vi "Oscilloscope.vi"() -> ()   [LabVIEW 2011]
uses:
  <vilib>/Analysis/5stat.llb/RMS (DBL).vi
  <vilib>/express/express analysis/Spectral/Block/exnSpectralBlock spectral measurements peak poly.vi
  <vilib>/express/express analysis/Spectral/Block/exnSpectralBlock spectral measurements peak DDT.vi
  <vilib>/express/express analysis/Spectral/XNode/ExpressSpectralMeasurementsBlockNode.xnode
  <vilib>/Analysis/NI_AALPro.lvlib
panel:
  in  "OK Button 3":bool
  out "Peak":dbl format="%#_3gV"
  in  "Duty Cycle (%)":dbl(knob)=50.0 scale=0.0..100.0
  out "Recorded Time":dbl format="%#.3f"
  in  "Save File":bool
  in  "Tab Control":enum32{"Waveform", "FFT"}(tab)
  out "Waveform":waveform(dbl)(graph) caption="Sine"
  in  "Position":ext(knob) scale=-5.0..5.0
  in  "OK Button":bool
  in  "Trigger":bool
  in  "Save Waveform":bool
  out "FFT":dynamicdata(graph) caption="FFT - (Peak)"
  in  "Scale":bool caption="Linear/Log"
  in  "FFT X reset":bool
  in  "Save FFT":bool
  in  "Offset RST":bool
  in  "Offset":dbl(knob) scale=-5.0..5.0
  out "Frequency":dbl format="%#_3pHz"
  out "Waveform 2":dynamicdata(graph) caption="DC with Uniform Noise"
  in  "Noise":dbl(knob)=0.6 caption="Noise amplitude" scale=0.0..5.0
  out "Sine":bool
  out "Square":bool
  out "Triangle":bool
  out "Sawtooth":bool
  out "DC":bool
  in  "Function":i32(knob) scale=0.0..4.0 scale format="%#_2g"
  in  "Frequency":dbl(knob)=10.1 scale=20.0..20000.0 scale format="%#5_2p"
  out "DC Voltage":dbl format="%#_3gV"
  out "Amplitude":dbl format="%#_3gV"
  in  "Amplitude":dbl(knob)=1.0 scale=0.0..10.0
  out "Cursor Diff":dbl format="%#_3gV"
  out "Cursor 2":dbl format="%#_3gV"
  out "Cursor 1":dbl format="%#_4gV"
  out "RMS":dbl format="%0.2fV"
  out "Peak-to-Peak":dbl format="%#_3gV"
  in  "Volts/Div":i32(knob) scale=0.0..4.0
  in  "ms/Div":i32(knob) scale=0.0..4.0 scale format="%#_2g"
  in  "stop":bool
  # "Oscilloscope"
  # "Function Generator"
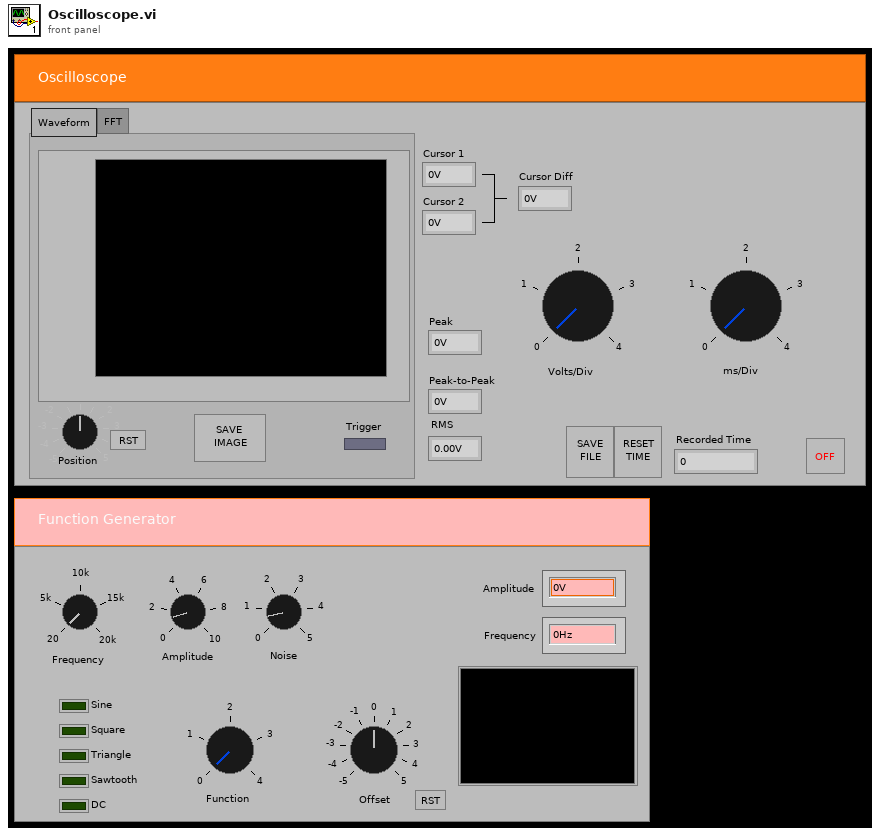
[diagram p1: front panel]
types:
  T1 = cluster{"averaging mode":u16, "weighting mode":u16, "number of averages":u32}
  T2 = cluster{"dB On (F)":bool, "unwrap phase (F)":bool, "convert to degree (F)":bool}
  T3 = typedef "imagedata.ctl" = cluster{"image type":i32, "image depth":i32, "image":u8[], "mask":u8[], "colors":u32[], "Rectangle":cluster{"left":i16, "top":i16, "right":i16, "bottom":i16}}
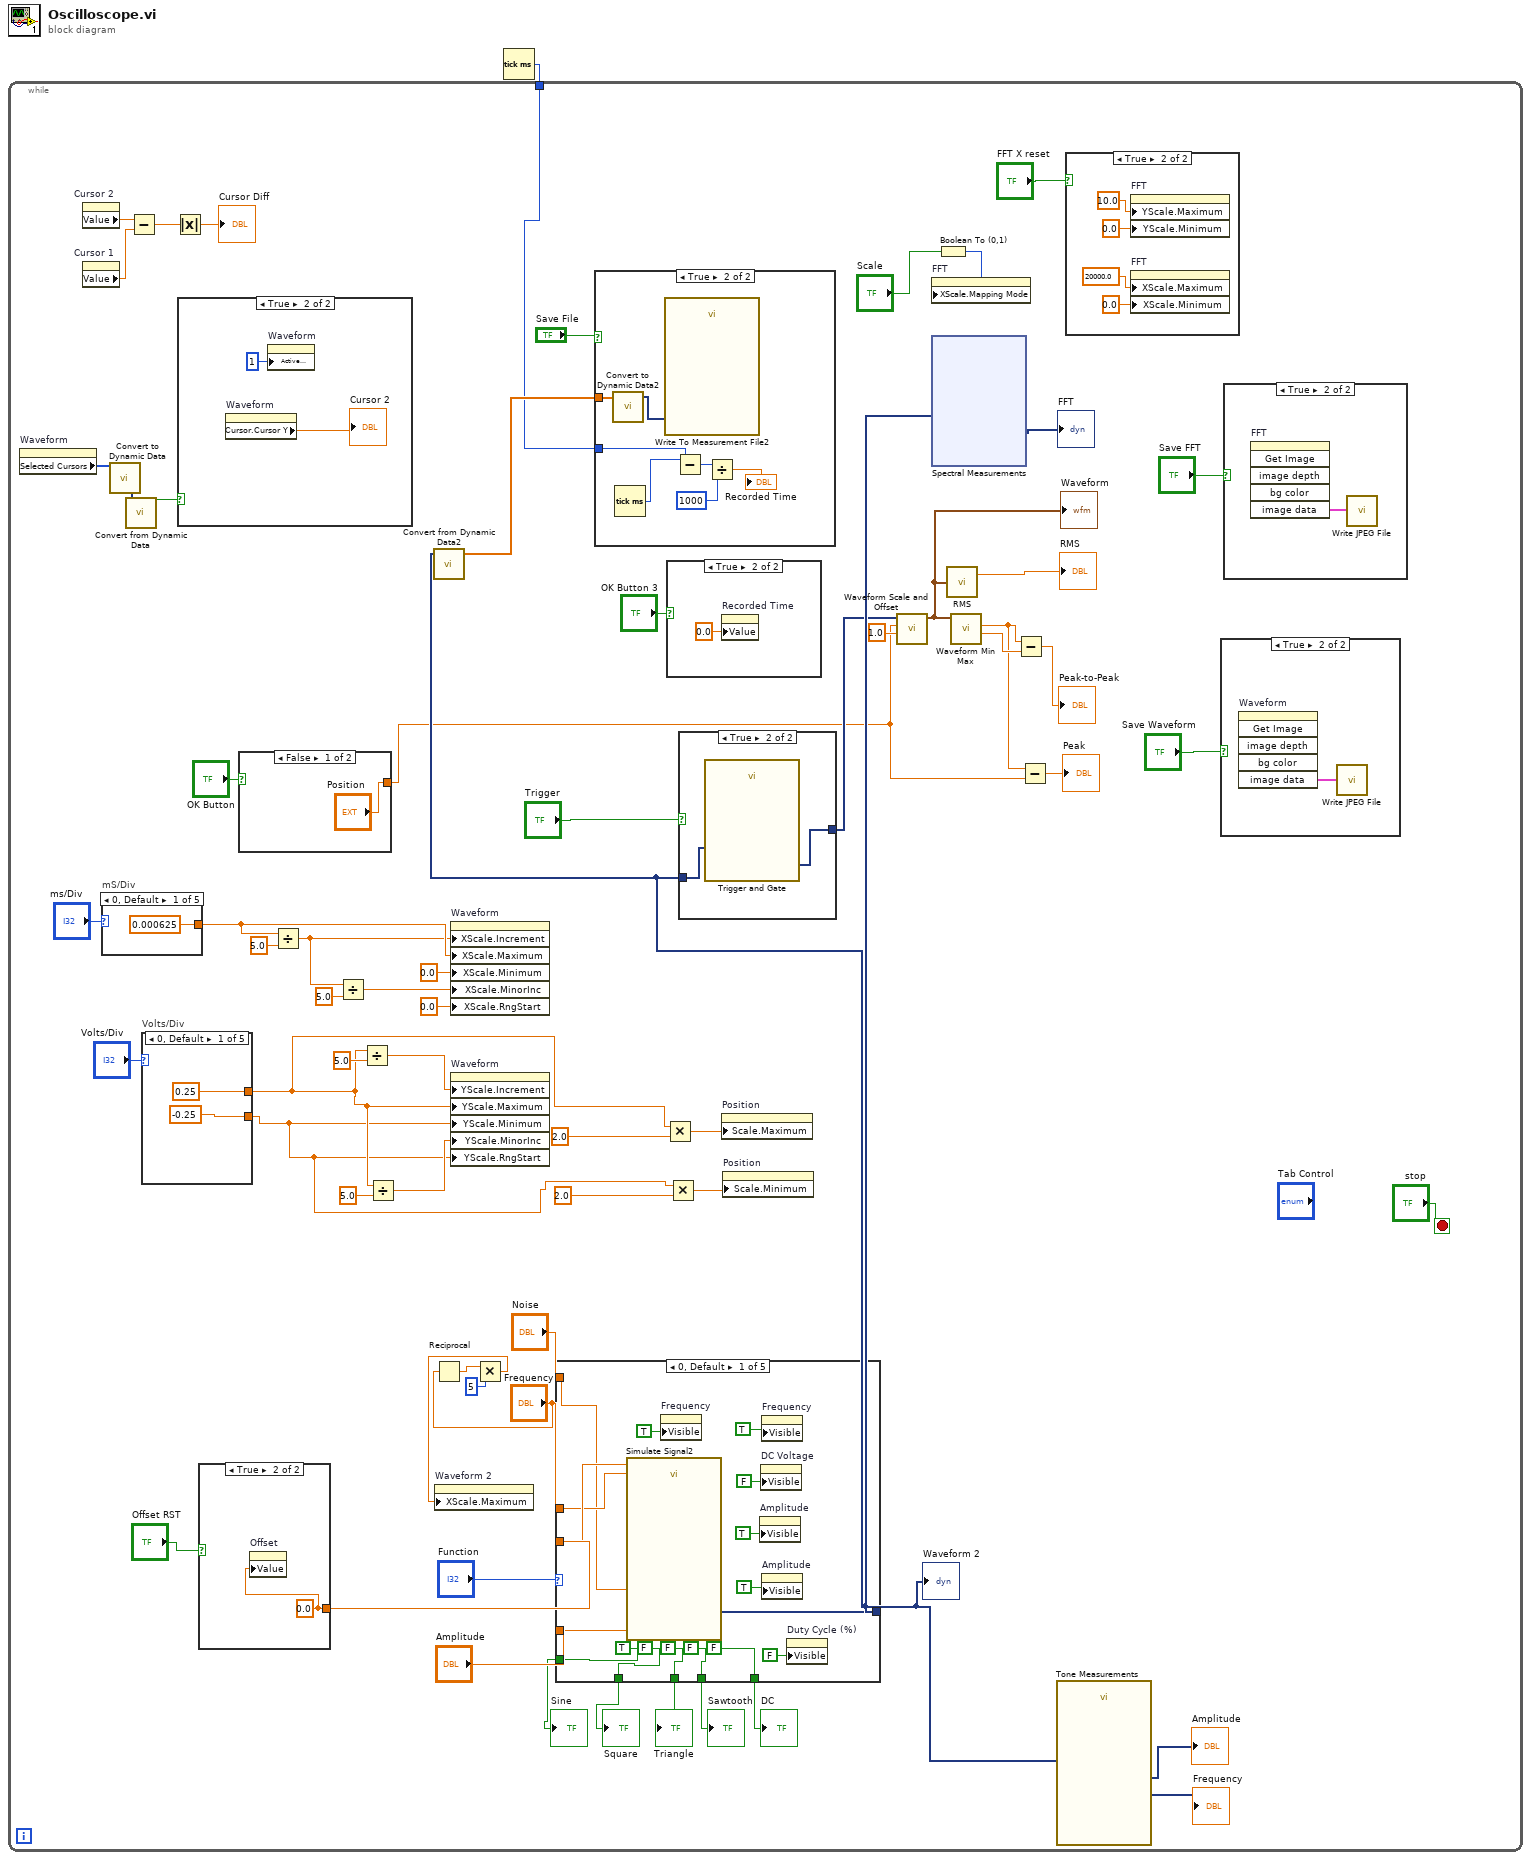
[diagram p0: block diagram]
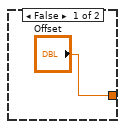
[diagram p7: hidden frame]
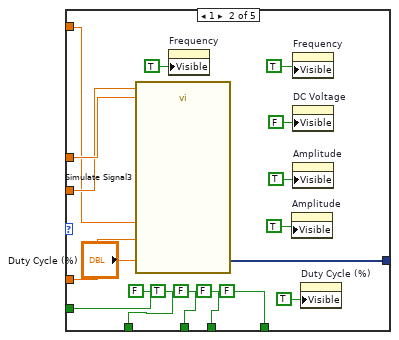
[diagram p8: hidden frame]
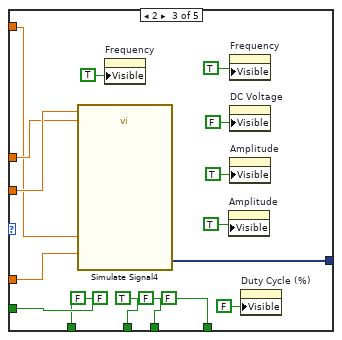
[diagram p9: hidden frame]
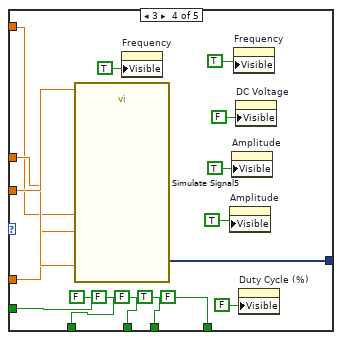
[diagram p10: hidden frame]
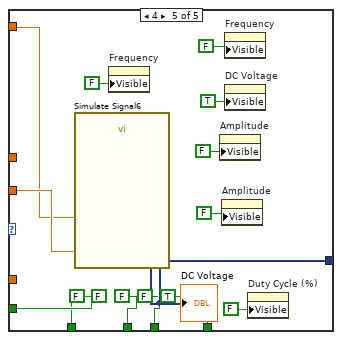
[diagram p11: hidden frame]
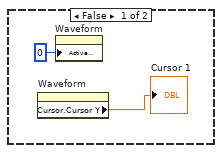
[diagram p13: hidden frame]
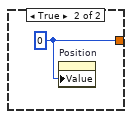
[diagram p14: hidden frame]
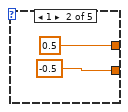
[diagram p15: hidden frame]
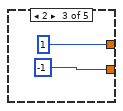
[diagram p16: hidden frame]
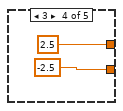
[diagram p17: hidden frame]
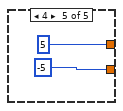
[diagram p18: hidden frame]
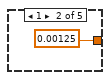
[diagram p19: hidden frame]
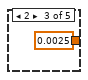
[diagram p20: hidden frame]
diagram:
  n1 = Tick Count (ms)() -> (millisecond timer value=w1:u32)
  n2 = while {
    tunnel: w1 -> [w13]
    stop <- "stop" stop-if-true
    n3 = property on="Waveform" class="WFGraph (strict)"() -> ("Selected Cursors"=w44:u32[])  [unwired: 2 in, 2 out]
    n4 = property on="Cursor 2" class="DigNum (strict)"() -> ("Value"=w48:dbl)  [unwired: 2 in, 2 out]
    n5 = property on="Cursor 1" class="DigNum (strict)"() -> ("Value"=w47:dbl)  [unwired: 2 in, 2 out]
    n6 = case "mS/Div" shown="0, Default" "ms/Div" {
      tunnel: [0.000625 0.00125 0.0025 0.005 0.01] -> w59
      frame 0, Default {
      }
      frame 1 {
      }
      frame 2 {
      }
      frame 3 {
      }
      frame 4 {
      }
    }
    n7 = call "Convert to Dynamic Data"("Array"=w44) -> ("Dynamic Data Type"=w43:dynamicdata)  [unwired: 3 in]
    n8 = call "Convert from Dynamic Data"("Dynamic Data Type"=w43) -> ("Scalar"=w42:bool)  [unwired: 3 in]
    n9 = Subtract(x=w48, y=w47) -> (x-y=w46:dbl)
    n10 = case "Volts/Div" shown="0, Default" "Volts/Div" {
      tunnel: [0.25 0.5 1 2.5 5] -> w36
      tunnel: [-0.25 -0.5 -1 -2.5 -5] -> w35
      frame 0, Default {
      }
      frame 1 {
      }
      frame 2 {
      }
      frame 3 {
      }
      frame 4 {
      }
    }
    n11 = Absolute Value(x=w46) -> (abs(x)=→"Cursor Diff":dbl)
    n12 = case shown="True" w42 {
      frame False {
        n13 = property on="Waveform" class="WFGraph (strict)"() -> ("Cursor.Cursor Y"=→"Cursor 1":dbl)  [unwired: 2 in, 2 out]
        n14 = property on="Waveform" class="WFGraph (strict)"("Active Cursor"=u32 0) -> ()  [unwired: 2 in, 2 out]
      }
      frame True {
        n15 = property on="Waveform" class="WFGraph (strict)"() -> ("Cursor.Cursor Y"=→"Cursor 2":dbl)  [unwired: 2 in, 2 out]
        n16 = property on="Waveform" class="WFGraph (strict)"("Active Cursor"=u32 1) -> ()  [unwired: 2 in, 2 out]
      }
    }
    n17 = case shown="True" "Offset RST" {
      tunnel: ["Offset" w92] -> w18
      frame False {
      }
      frame True {
        w92 = 0.0 ("Offset")
        n18 = property on="Offset" class="Knob (strict)"("Value"=w92) -> ()  [unwired: 2 in, 2 out]
      }
    }
    n19 = case shown="False" "OK Button" {
      tunnel: ["Position" w180] -> w7
      frame False {
      }
      frame True {
        w180 = 0
        n20 = property on="Position" class="Knob (strict)"("Value"=w180) -> ()  [unwired: 2 in, 2 out]
      }
    }
    n21 = Divide(x=w59, y=5.0) -> (x/y=w58:dbl)
    n22 = Divide(x=w58, y=5.0) -> (x/y=w57:dbl)
    n23 = Divide(x=w36, y=5.0) -> (x/y=w51:dbl)
    n24 = Divide(x=w36, y=5.0) -> (x/y=w49:dbl)
    n25 = Reciprocal(x="Frequency") -> (1/x=w28:dbl)
    n26 = property on="Waveform" class="WFGraph (strict)"("XScale.Increment"=w58, "XScale.Maximum"=w59, "XScale.Minimum"=0.0 ("X Scale.Range:Minimum"), "XScale.MinorInc"=w57, "XScale.RngStart"=0.0 ("X Scale.Range:Start")) -> ()  [unwired: 2 in, 2 out]
    n27 = property on="Waveform" class="WFGraph (strict)"("YScale.Increment"=w51, "YScale.Maximum"=w36, "YScale.Minimum"=w35, "YScale.MinorInc"=w49, "YScale.RngStart"=w35) -> ()  [unwired: 2 in, 2 out]
    n28 = Multiply(x=w28, y=5) -> (x*y=w27:dbl)
    n29 = property on="Waveform 2" class="WFGraph (strict)"("XScale.Maximum"=w27) -> ()  [unwired: 2 in, 2 out]
    n30 = case shown="0, Default" "Function" {
      tunnel: w18 -> [w108 w124 w141 w157 w170]
      tunnel: "Amplitude" -> [w107 w123 w139 w155 _]
      tunnel: [w106 w122 w138 w154 w171] -> w12
      tunnel: "Frequency" -> [w105 w125 w140 w156 _]
      tunnel: "Noise" -> [w104 w121 w137 w153 w169]
      tunnel: [TRUE FALSE FALSE FALSE FALSE] -> w25
      tunnel: [FALSE TRUE FALSE FALSE FALSE] -> w24
      tunnel: [FALSE FALSE TRUE FALSE FALSE] -> w23
      tunnel: [FALSE FALSE FALSE TRUE FALSE] -> w22
      tunnel: [FALSE FALSE FALSE FALSE TRUE] -> w21
      frame 0, Default {
        n31 = call "Simulate Signal2"("Offset"=w108, "Frequency"=w105, "Amplitude"=w107, "Noise amplitude"=w104) -> ("Sine with Uniform Noise"=w106:dynamicdata)  [unwired: 10 in, 1 out]
        n32 = property on="Frequency" class="Knob (strict)"("Visible"=TRUE) -> ()  [unwired: 2 in, 2 out]
        n33 = property on="Amplitude" class="DigNum (strict)"("Visible"=TRUE) -> ()  [unwired: 2 in, 2 out]
        n34 = property on="DC Voltage" class="DigNum (strict)"("Visible"=FALSE) -> ()  [unwired: 2 in, 2 out]
        n35 = property on="Frequency" class="DigNum (strict)"("Visible"=TRUE) -> ()  [unwired: 2 in, 2 out]
        n36 = property on="Amplitude" class="Knob (strict)"("Visible"=TRUE) -> ()  [unwired: 2 in, 2 out]
        n37 = property on="Duty Cycle (%)" class="Knob (strict)"("Visible"=FALSE) -> ()  [unwired: 2 in, 2 out]
      }
      frame 1 {
        n38 = call "Simulate Signal3"("Offset"=w124, "Duty Cycle (%)"="Duty Cycle (%)", "Frequency"=w125, "Amplitude"=w123, "Noise amplitude"=w121) -> ("Square with Uniform Noise"=w122:dynamicdata)  [unwired: 9 in, 1 out]
        n39 = property on="Frequency" class="Knob (strict)"("Visible"=TRUE) -> ()  [unwired: 2 in, 2 out]
        n40 = property on="Amplitude" class="Knob (strict)"("Visible"=TRUE) -> ()  [unwired: 2 in, 2 out]
        n41 = property on="Frequency" class="DigNum (strict)"("Visible"=TRUE) -> ()  [unwired: 2 in, 2 out]
        n42 = property on="DC Voltage" class="DigNum (strict)"("Visible"=FALSE) -> ()  [unwired: 2 in, 2 out]
        n43 = property on="Amplitude" class="DigNum (strict)"("Visible"=TRUE) -> ()  [unwired: 2 in, 2 out]
        n44 = property on="Duty Cycle (%)" class="Knob (strict)"("Visible"=TRUE) -> ()  [unwired: 2 in, 2 out]
      }
      frame 2 {
        n45 = call "Simulate Signal4"("Offset"=w141, "Frequency"=w140, "Amplitude"=w139, "Noise amplitude"=w137) -> ("Triangle with Uniform Noise"=w138:dynamicdata)  [unwired: 10 in, 1 out]
        n46 = property on="Frequency" class="Knob (strict)"("Visible"=TRUE) -> ()  [unwired: 2 in, 2 out]
        n47 = property on="Amplitude" class="Knob (strict)"("Visible"=TRUE) -> ()  [unwired: 2 in, 2 out]
        n48 = property on="Frequency" class="DigNum (strict)"("Visible"=TRUE) -> ()  [unwired: 2 in, 2 out]
        n49 = property on="DC Voltage" class="DigNum (strict)"("Visible"=FALSE) -> ()  [unwired: 2 in, 2 out]
        n50 = property on="Amplitude" class="DigNum (strict)"("Visible"=TRUE) -> ()  [unwired: 2 in, 2 out]
        n51 = property on="Duty Cycle (%)" class="Knob (strict)"("Visible"=FALSE) -> ()  [unwired: 2 in, 2 out]
      }
      frame 3 {
        n52 = call "Simulate Signal5"("Offset"=w157, "Frequency"=w156, "Amplitude"=w155, "Noise amplitude"=w153) -> ("Sawtooth with Uniform Noise"=w154:dynamicdata)  [unwired: 10 in, 1 out]
        n53 = property on="Frequency" class="Knob (strict)"("Visible"=TRUE) -> ()  [unwired: 2 in, 2 out]
        n54 = property on="Amplitude" class="Knob (strict)"("Visible"=TRUE) -> ()  [unwired: 2 in, 2 out]
        n55 = property on="Amplitude" class="DigNum (strict)"("Visible"=TRUE) -> ()  [unwired: 2 in, 2 out]
        n56 = property on="Frequency" class="DigNum (strict)"("Visible"=TRUE) -> ()  [unwired: 2 in, 2 out]
        n57 = property on="DC Voltage" class="DigNum (strict)"("Visible"=FALSE) -> ()  [unwired: 2 in, 2 out]
        n58 = property on="Duty Cycle (%)" class="Knob (strict)"("Visible"=FALSE) -> ()  [unwired: 2 in, 2 out]
      }
      frame 4 {
        n59 = call "Simulate Signal6"("Offset"=w170, "Noise amplitude"=w169) -> ("DC with Uniform Noise"=w171:dynamicdata)  [unwired: 12 in, 1 out]
        "DC Voltage" <- w171
        n60 = property on="Frequency" class="Knob (strict)"("Visible"=FALSE) -> ()  [unwired: 2 in, 2 out]
        n61 = property on="Amplitude" class="DigNum (strict)"("Visible"=FALSE) -> ()  [unwired: 2 in, 2 out]
        n62 = property on="Amplitude" class="Knob (strict)"("Visible"=FALSE) -> ()  [unwired: 2 in, 2 out]
        n63 = property on="Frequency" class="DigNum (strict)"("Visible"=FALSE) -> ()  [unwired: 2 in, 2 out]
        n64 = property on="DC Voltage" class="DigNum (strict)"("Visible"=TRUE) -> ()  [unwired: 2 in, 2 out]
        n65 = property on="Duty Cycle (%)" class="Knob (strict)"("Visible"=FALSE) -> ()  [unwired: 2 in, 2 out]
      }
    }
    "DC" <- w21
    "Sawtooth" <- w22
    "Triangle" <- w23
    "Square" <- w24
    "Sine" <- w25
    "Waveform 2" <- w12
    n66 = call "Convert from Dynamic Data2"("Dynamic Data Type"=w12) -> ("Array"=w14:dbl[])  [unwired: 3 in]
    n67 = case shown="True" "Save File" {
      tunnel: w14 -> [_ w80]
      tunnel: w13 -> [_ w75]
      frame False {
      }
      frame True {
        n68 = call "Convert to Dynamic Data2"("Array"=w80) -> ("Dynamic Data Type"=w79:dynamicdata)  [unwired: 3 in]
        n69 = Tick Count (ms)() -> (millisecond timer value=w76:u32)
        n70 = call "Write To Measurement File2"("Signals"=w79) -> ()  [unwired: 16 in, 3 out]
        n71 = Subtract(x=w76, y=w75) -> (x-y=w74:u32)
        n72 = Divide(x=w74, y=u32 1000) -> (x/y=→"Recorded Time":dbl)
      }
    }
    n73 = Multiply(x=w36, y=2.0) -> (x*y=w40:dbl)
    n74 = case shown="True" "OK Button 3" {
      frame False {
      }
      frame True {
        n75 = property on="Recorded Time" class="DigNum (strict)"("Value"=0.0 ("Recorded Time")) -> ()  [unwired: 2 in, 2 out]
      }
    }
    n76 = Multiply(x=w35, y=2.0) -> (x*y=w39:dbl)
    n77 = case shown="True" "Trigger" {
      tunnel: [w172 w174] -> w8
      tunnel: w12 -> [w172 w173]
      frame False {
      }
      frame True {
        n78 = call "Trigger and Gate"("Signals"=w173) -> ("Triggered Signals"=w174:dynamicdata)  [unwired: 7 in, 3 out]
      }
    }
    n79 = property on="Position" class="Knob (strict)"("Scale.Maximum"=w40) -> ()  [unwired: 2 in, 2 out]
    n80 = property on="Position" class="Knob (strict)"("Scale.Minimum"=w39) -> ()  [unwired: 2 in, 2 out]
    n81 = call <vilib>:"Waveform Scale and Offset.vi"("scale"=1.0, "offset"=w7, "waveform in"=w8) -> ("waveform out"=w34:waveform(dbl))  [unwired: 7 in, 1 out]
    "Waveform" <- w34
    n82 = xnode "Spectral Measurements"("Signals"=w12) -> ("FFT - (Peak)"=→"FFT":dynamicdata)  [unwired: 1 in, 2 out]
    n83 = Boolean To (0,1)(Boolean="Scale") -> (0, 1=w10:i16)
    n84 = property on="FFT" class="WFGraph (strict)"("XScale.Mapping Mode"=w10) -> ()  [unwired: 2 in, 2 out]
    n85 = call-poly <vilib>:"RMS.vi"("X"=w34) -> ("rms value"=→"RMS":dbl)  [unwired: 1 out]
    n86 = call <vilib>:"Waveform Min Max.vi"("waveform in"=w34) -> ("Y min"=w55:dbl, "Y max"=w5:dbl)  [unwired: 5 in, 4 out]
    n87 = Subtract(x=w5, y=w55) -> (x-y=→"Peak-to-Peak":dbl)
    n88 = Subtract(x=w5, y=w7) -> (x-y=→"Peak":ext)
    n89 = call "Tone Measurements"("Signals"=w12) -> ("Frequency"=→"Frequency":dynamicdata, "Amplitude"=→"Amplitude":dynamicdata)  [unwired: 8 in, 1 out]
    n90 = case shown="True" "FFT X reset" {
      frame False {
      }
      frame True {
        n91 = property on="FFT" class="WFGraph (strict)"("YScale.Maximum"=10.0 ("Y Scale.Range:Maximum"), "YScale.Minimum"=0.0 ("Y Scale.Range:Minimum")) -> ()  [unwired: 2 in, 2 out]
        n92 = property on="FFT" class="WFGraph (strict)"("XScale.Maximum"=20000.0 ("X Scale.Range:Maximum"), "XScale.Minimum"=0.0 ("X Scale.Range:Minimum")) -> ()  [unwired: 2 in, 2 out]
      }
    }
    n93 = case shown="True" "Save Waveform" {
      frame False {
      }
      frame True {
        n94 = invoke on="Waveform" class="WFGraph (strict)" method="Get Image"() -> ("image data"=w69:T3)  [unwired: 6 in, 5 out]
        n95 = call <vilib>:"Write JPEG File.vi"("image data"=w69) -> ()  [unwired: 9 in, 2 out]
      }
    }
    n96 = case shown="True" "Save FFT" {
      frame False {
      }
      frame True {
        n97 = invoke on="FFT" class="WFGraph (strict)" method="Get Image"() -> ("image data"=w68:T3)  [unwired: 6 in, 5 out]
        n98 = call <vilib>:"Write JPEG File.vi"("image data"=w68) -> ()  [unwired: 9 in, 2 out]
      }
    }
  }
